vi "Load I16 image data for single image from TIF stack file.vi"(8 "error in":errorcluster, 9 "DirEntries":T2[](array[typedef]), 10 "Litt/BigEnd":bool, 11 "File":refnum<file>) -> (0 "error out":errorcluster, 1 "Gray16":i16[][](array[numeric]), 3 "File":refnum<file>)   [LabVIEW 2013, in "Tiff reader.lvlib"]
doc: "Read I16 image data from a TIF stack."
uses:
  Tiff reader.lvlib
  IFD Entry.ctl
  FieldTypes.ctl
panel:
  out "N_Bits":u64
  out "PhotoM":T1(ring)=enum."BlackIsZero"
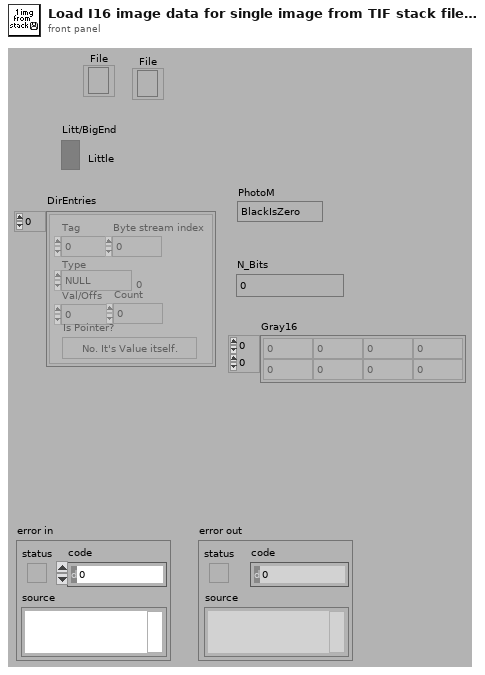
[diagram p1: front panel]
types:
  T1 = enum16{"WhiteIsZero", "BlackIsZero", "RGB", "RGBPalette", "TranspMask", "CMYK", "YCbCr", "Null", "CIELab"}
  T2 = typedef "Tiff reader.lvlib/IFD Entry.ctl" = cluster{"Tag":u16, "Type":T3, "Count":u32, "Val/Offs":u32, "Is Pointer?":bool, "Byte stream index":i32}
  T3 = typedef "Tiff reader.lvlib/FieldTypes.ctl" = enum16{"NULL", "U8", "ASCII7", "U16", "U32", "RATIONAL", "SByte(I8)", "Undef(8Bit)", "I16", "I32", "SRat(4B:4B)", "SGL(4Byte)", "DBL(8Byte)"}
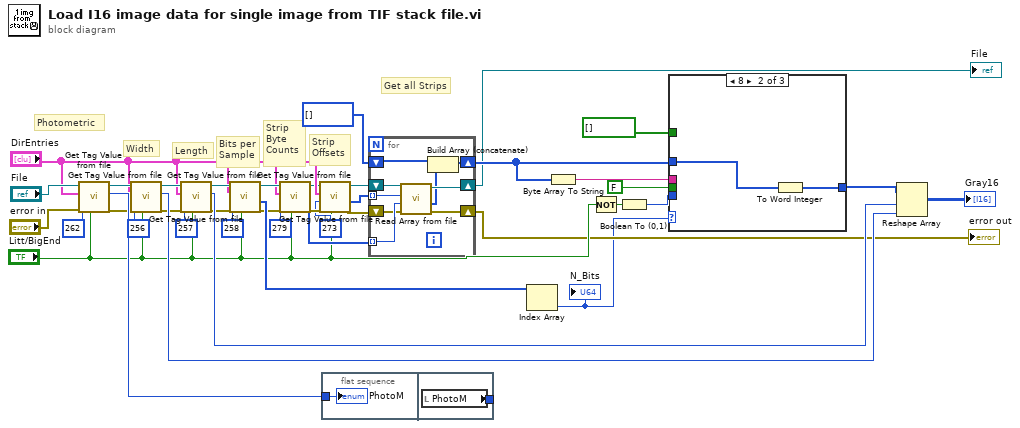
[diagram p0: block diagram]
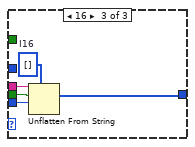
[diagram p3: hidden frame]
diagram:
  # "Get all Strips"
  # "Strip\nOffsets"
  # "Strip\nByte\nCounts"
  # "Bits per\nSample"
  # "Photometric"
  # "Length"
  # "Width"
  n1 = call "Get Tag Value from file.vi"("Litt/BigEnd"="Litt/BigEnd", "error in"="error in", "Tag Code"=u16 262, "DirEntries"="DirEntries", "File"="File") -> ("error out"=w33:errorcluster, "Single Value"=w35:u32, "File"=w18:refnum<file>)  [unwired: 4 out]
  n2 = call "Get Tag Value from file.vi"("Litt/BigEnd"="Litt/BigEnd", "error in"=w33, "Tag Code"=u16 256, "DirEntries"="DirEntries", "File"=w18) -> ("error out"=w30:errorcluster, "Single Value"=w34:u32, "File"=w17:refnum<file>)  [unwired: 4 out]
  n3 = call "Get Tag Value from file.vi"("Litt/BigEnd"="Litt/BigEnd", "error in"=w30, "Tag Code"=u16 257, "DirEntries"="DirEntries", "File"=w17) -> ("error out"=w26:errorcluster, "Single Value"=w31:u32, "File"=w27:refnum<file>)  [unwired: 4 out]
  n4 = call "Get Tag Value from file.vi"("Litt/BigEnd"="Litt/BigEnd", "error in"=w26, "Tag Code"=u16 258, "DirEntries"="DirEntries", "File"=w27) -> ("error out"=w22:errorcluster, "Multiple Values"=w28:u64[], "File"=w24:refnum<file>)  [unwired: 4 out]
  n5 = call "Get Tag Value from file.vi"("Litt/BigEnd"="Litt/BigEnd", "error in"=w22, "Tag Code"=u16 279, "DirEntries"="DirEntries", "File"=w24) -> ("error out"=w19:errorcluster, "Multiple Values"=w23:u64[], "File"=w15:refnum<file>)  [unwired: 4 out]
  n6 = call "Get Tag Value from file.vi"("Litt/BigEnd"="Litt/BigEnd", "error in"=w19, "Tag Code"=u16 273, "DirEntries"="DirEntries", "File"=w15) -> ("error out"=w11:errorcluster, "Multiple Values"=w20:u64[], "File"=w12:refnum<file>)  [unwired: 4 out]
  n7 = flat-sequence {
    tunnel: w35 -> [w41]
    tunnel: [w42] -> _
    frame #0 {
      "PhotoM" <- w41
    }
    frame #1 {
      n8 = local read "PhotoM"() -> (w42:T1)
    }
  }
  n9 = for {
    tunnel: w20 -> [w49] mode=indexing
    tunnel: w23 -> [w48] mode=indexing
    shift-right: [w51] -> w39
    shift-left: u8[] [] -> [w50]
    shift-right: [w46] -> w9
    shift-left: w12 -> [w47]
    shift-right: [w44] -> w10
    shift-left: w11 -> [w43]
    n10 = call "Read Array from file.vi"("error in"=w43, "bytes to read"=w48, "File location in"=w49, "File"=w47) -> ("error out"=w44:errorcluster, "Array of U8s"=w45:u8[], "File out"=w46:refnum<file>)  [unwired: 1 out]
    n11 = Build Array (concatenate)(w50, w45) -> (w51:u8[])
  }
  "File" <- w9
  "error out" <- w10
  n12 = Index Array(array=w28) -> (element=w3:u64)  [unwired: 1 in]
  "N_Bits" <- w3
  n13 = Byte Array To String(unsigned byte array=w39) -> (string=w8:string)
  n14 = Not(x="Litt/BigEnd") -> (.not. x?=w5:bool)
  n15 = Boolean To (0,1)(Boolean=w5) -> (0, 1=w6:i16)
  n16 = case shown="8" w3 {
    tunnel: w8 -> [_ _ w58]
    tunnel: [_ w52 w54] -> w4
    tunnel: FALSE ("data includes array or string size? (T)") -> [_ _ w57]
    tunnel: w6 -> [_ _ w56]
    tunnel: w39 -> [_ w53 _]
    tunnel: bool[] [] -> [_ _ _]
    frame 0, 4, Default {
      # "not\nsupported"
    }
    frame 8 {
      n17 = To Word Integer(number=w53) -> (16bit integer=w52:i16[])
    }
    frame 16 {
      w55 = i16[] []  # I16
      n18 = Unflatten From String(type=w55, binary string=w58, data includes array or string size? (T)=w57, byte order (0:big-endian, network order)=w56) -> (value=w54:i16[])  [unwired: 1 in, 2 out]
    }
  }
  n19 = Reshape Array(w4, w31, w34) -> (→"Gray16":i16[][])
